vi "NaN entfernen.vi"(10 "Messdaten":sgl[](array[numeric])) -> (2 "Messdaten":sgl[](array[numeric]))   [LabVIEW 2020, in "Messdaten.lvlib"]
uses:
  Messdaten.lvlib
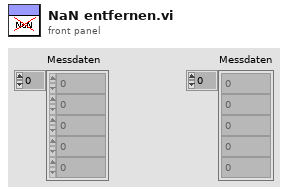
[diagram p1: front panel]
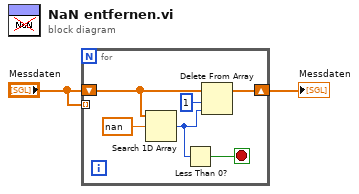
[diagram p0: block diagram]
diagram:
  n1 = for {
    shift-right: [w5] -> w2
    shift-left: "Messdaten" -> [w7]
    tunnel: "Messdaten" -> [_] mode=indexing
    stop <- w3 stop-if-true
    n2 = Search 1D Array(1D array=w7, element=sgl nan ("Element")) -> (index of element=w4:i32)  [unwired: 1 in]
    n3 = Less Than 0?(x=w4) -> (x < 0?=w3:bool)
    n4 = Delete From Array(array=w7, length=1 ("Länge"), index=w4) -> (array with subset deleted=w5:sgl[])  [unwired: 1 out]
  }
  "Messdaten" <- w2
